vi "Run All.vi"(8 "error in (no error)":errorcluster, 11 "Runnable In":refnum<class "Runnable.lvclass">) -> (0 "error out":errorcluster, 2 "Results":T1[](array[typedef]))   [LabVIEW 2020, in "Runnable.lvclass"]
uses:
  Runnable.lvclass
  Result/Status.ctl
  Result/Result.lvlib
  Result/Type.ctl
  Result/Result.ctl
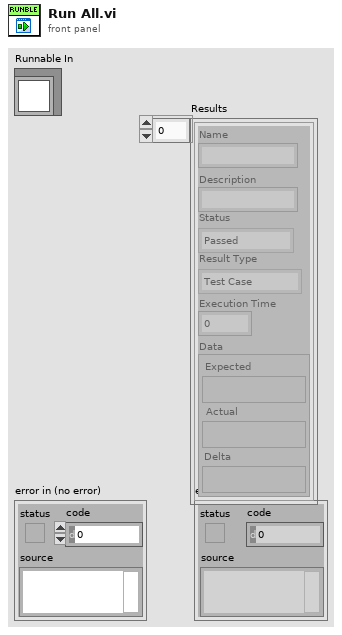
[diagram p1: front panel]
types:
  T1 = typedef "Result.lvlib/Result.ctl" = cluster{"Name":string, "Description":string, "Status":T2, "Result Type":T3, "Execution Time":dbl, "Data":cluster{"Expected":variant, "Actual":variant, "Delta":variant}}
  T2 = typedef "Result.lvlib/Status.ctl" = enum16{"", "Passed", "Failed", "Error", "Skipped", "Setup Error", "Broken", "Teardown Error"}
  T3 = typedef "Result.lvlib/Type.ctl" = enum16{"Test Case", "Test Suite", "Test Run", "Pass", "Fail", "Skip", "Pass if", "Fail if", "Pass if Error", "Fail if Error", "Pass if Equal", "Fail if Equal"}
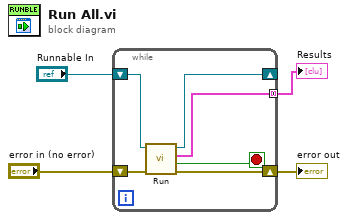
[diagram p0: block diagram]
diagram:
  n1 = while {
    tunnel: [w7] -> w1 mode=concatenating
    shift-right: [w9] -> w3
    shift-left: "error in (no error)" -> [w10]
    shift-right: [w6] -> _
    shift-left: "Runnable In" -> [w8]
    stop <- w5 stop-if-true
    n2 = call-dynamic "Run.vi"("error in (no error)"=w10, "Runnable In"=w8) -> ("error out"=w9:errorcluster, "Done?"=w5:bool, "Results"=w7:T1[], "Runnable Out"=w6:refnum<class "Runnable.lvclass">)  [unwired: 6 in]
  }
  "error out" <- w3
  "Results" <- w1
